vi "PictureDisplay.vi"(8 "error In":errorcluster, 9 "ImagesFolderPath":path=path "../../Config/Images", 10 "Image Array":string[](array[string])=["Test1", "Test2", "Test3"], 11 "Sequence Context":refnum<k7>) -> (0 "error out":errorcluster)   [LabVIEW 2021]
doc: "Use this template to display pictures of the step to execute. For detail information refer to the block diagram."
uses:
  <vilib>/addons/TestStand/_TSUtility.llb/TestStand - Start Modal Dialog (Sequence Context).vi
  <vilib>/addons/TestStand/_TSUtility.llb/TestStand - End Modal Dialog (Sequence Context).vi
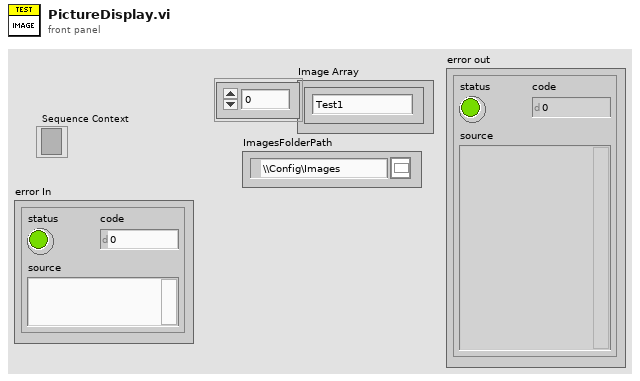
[diagram p1: front panel]
types:
  T1 = typedef "imagedata.ctl" = cluster{"image type":i32, "image depth":i32, "image":u8[], "mask":u8[], "colors":u32[], "Rectangle":cluster{"left":i16, "top":i16, "right":i16, "bottom":i16}}
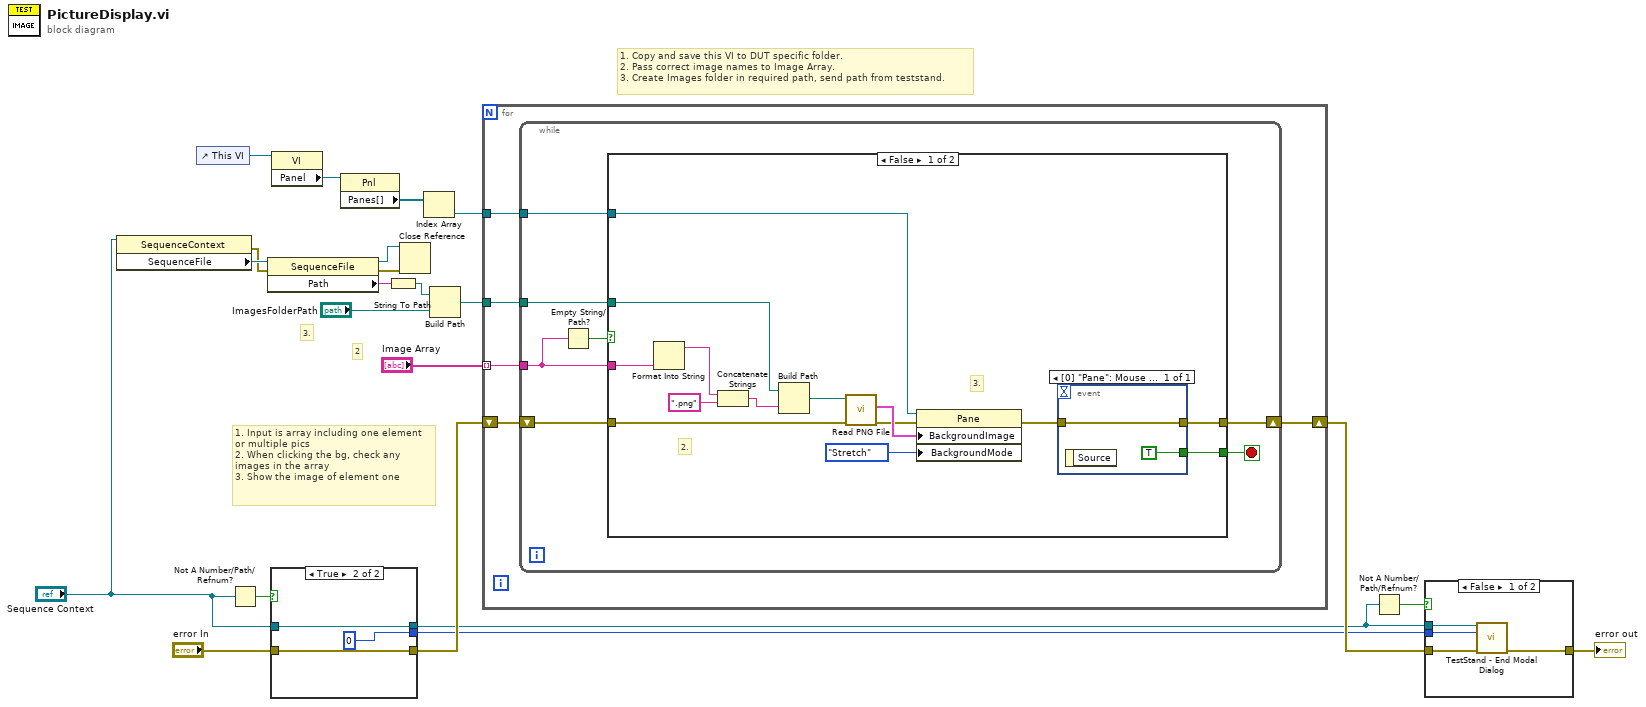
[diagram p0: block diagram]
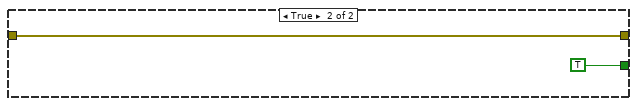
[diagram p2: hidden frame]
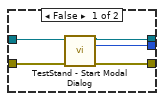
[diagram p3: hidden frame]
diagram:
  # "3."
  # "2"
  # "1. Copy and save this VI to DUT specific folder.\n2. Pass correct image names to Image Array.\n3. Create Images folder in required path, send path from teststand."
  # "1. Input is array including one element or multiple pics\n2. When clicking the bg, check any images in the array  \n3. Show the image of element one"
  n1 = property class="SequenceContext"(reference="Sequence Context") -> (error out=w8:errorcluster, "SequenceFile"=w9:refnum<k7>)  [unwired: 1 in, 1 out]
  n2 = control-ref of="This VI"() -> (w13:refnum<vi>)
  n3 = Not A Number/Path/Refnum?(number/path/refnum="Sequence Context") -> (NaN/Path/Refnum?=w22:bool)
  n4 = property class="SequenceFile"(reference=w9, error in=w8) -> (reference out=w3:refnum<k7>, error out=w4:errorcluster, "Path"=w7:string)
  n5 = case shown="True" w22 {
    tunnel: "error In" -> [w25 w30]
    tunnel: [w24 w30] -> w18
    tunnel: "Sequence Context" -> [w23 w28]
    tunnel: [w27 w28] -> w16
    tunnel: [w26 0 ("Modal ID")] -> w15
    frame False {
      n6 = call-poly <vilib>:"TestStand - Start Modal Dialog.vi"("Sequence Context In"=w23, "error in (no error)"=w25) -> ("Sequence Context Out"=w27:refnum<k7>, "Modal ID"=w26:i32, "error out"=w24:errorcluster)  [unwired: 9 in, 2 out]
    }
    frame True {
    }
  }
  n7 = property class="VI"(reference=w13) -> ("Panel"=w12:refnum<vi>)  [unwired: 1 in, 2 out]
  n8 = property class="Pnl"(reference=w12) -> ("Panes[]"=w11:refnum<vi>[])  [unwired: 1 in, 2 out]
  n9 = String To Path(string=w7) -> (path=w6:path)
  n10 = Close Reference(reference=w3, error in (no error)=w4) -> ()  [unwired: 1 out]
  n11 = Index Array(array=w11) -> (element=w10:refnum<vi>)  [unwired: 1 in]
  n12 = Build Path(base path=w6, name or relative path="ImagesFolderPath") -> (appended path=w2:path)
  n13 = for {
    tunnel: w2 -> [w33]
    tunnel: "Image Array" -> [w32] mode=indexing
    shift-right: [w34] -> w17
    shift-left: w18 -> [w35]
    tunnel: w10 -> [w31]
    n14 = while {
      tunnel: w33 -> [w40]
      tunnel: w32 -> [w39]
      tunnel: w31 -> [w37]
      shift-right: [w41] -> w34
      shift-left: w35 -> [w42]
      stop <- w36 stop-if-true
      n15 = Empty String/Path?(string/path=w39) -> (empty?=w38:bool)
      n16 = case shown="False" w38 {
        tunnel: w42 -> [w56 w60]
        tunnel: [w44 w60] -> w41
        tunnel: w40 -> [w55 _]
        tunnel: w39 -> [w54 _]
        tunnel: w37 -> [w46 _]
        tunnel: [w43 TRUE] -> w36
        frame False {
          # "3."
          # "2."
          n17 = Format Into String(w54) -> (resulting string=w47:string)  [unwired: 3 in, 1 out]
          n18 = Concatenate Strings(w47, ".png" ("string")) -> (w50:string)
          n19 = Build Path(base path=w55, name or relative path=w50) -> (appended path=w53:path)
          n20 = call <vilib>:"Read PNG File.vi"("error in (no error)"=w56, "path to PNG file"=w53) -> ("error out"=w48:errorcluster, "image data"=w52:T1)  [unwired: 7 in, 1 out]
          n21 = property class="Pane"(reference=w46, error in=w48, "BackgroundImage"=w52, "BackgroundMode"=enum16{"Stretch", "Center", "Tile"}."Stretch" ("Background Mode")) -> (error out=w45:errorcluster)  [unwired: 1 out]
          n22 = event shown="[0] \"Pane\": Mouse Up" {
            selector: _ -> [_]
            dyn-events: _ -> [_]
            timeout: _ -> [_]
            tunnel: w45 -> [w58]
            tunnel: [w58] -> w44
            tunnel: [TRUE] -> w43
            event Mouse Up {
              n23 = event-data() -> ()  [unwired: 1 in, 1 out]
            }
          }
        }
        frame True {
        }
      }
    }
  }
  n24 = Not A Number/Path/Refnum?(number/path/refnum=w16) -> (NaN/Path/Refnum?=w20:bool)
  n25 = case shown="False" w20 {
    tunnel: w17 -> [w64 w65]
    tunnel: w15 -> [w63 _]
    tunnel: [w61 w65] -> w19
    tunnel: w16 -> [w62 _]
    frame False {
      n26 = call-poly <vilib>:"TestStand - End Modal Dialog.vi"("Sequence Context In"=w62, "Modal ID"=w63, "error in (no error)"=w64) -> ("error out"=w61:errorcluster)  [unwired: 12 in]
    }
    frame True {
    }
  }
  "error out" <- w19
